vi "UTF8 Encoding to Unicode (UCS32).vi"(8 "error in":errorcluster, 9 "[UTF-8]":u8[](array[numeric])=[65, 226, 137, 162, 206, 145, 46, 237, 149, 156, 234, 189, 173, 236, 150, 180, 230, 151, 165, 230, 156, 172, 232, 170, 158, 240, 163, 142, 180] format="%.0x") -> (0 "error out":errorcluster, 1 "[UCS 32]":u32[](array[numeric]) format="%.0x", 4 "UCS 32":u32 format="%.0x")   [LabVIEW 2011]
doc: "Converts the given UTF-8 Encoded Unicode to UCS 32 Bit Representation of Unicode.\n\nUTF-8 is one of the Encodings to store the 21 bit Unicode numbers in a compact format.\n i.e. it stores the Unicode in one or more Byte sequences."
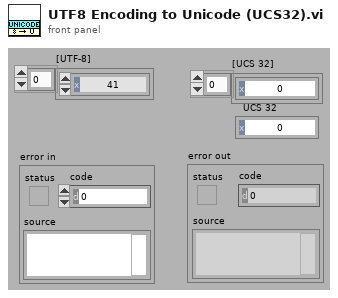
[diagram p1: front panel]
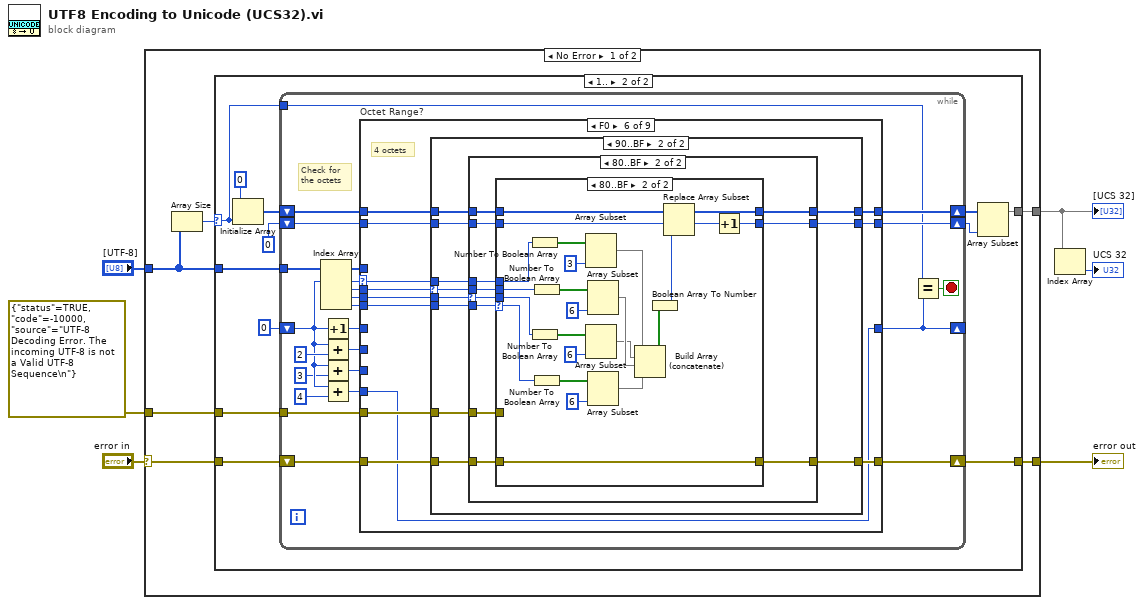
[diagram p0: block diagram]
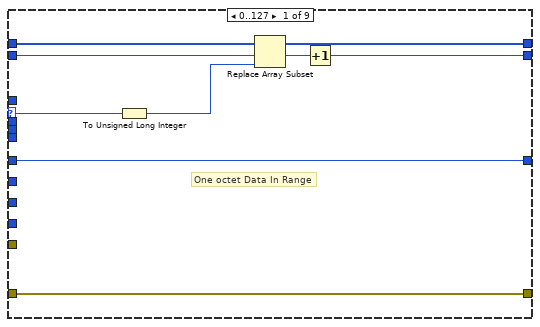
[diagram p3: hidden frame]
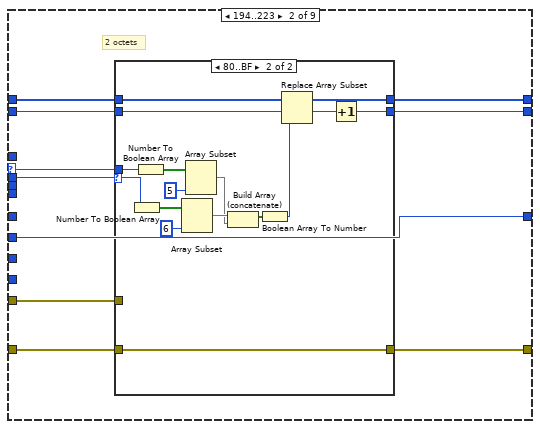
[diagram p4: hidden frame]
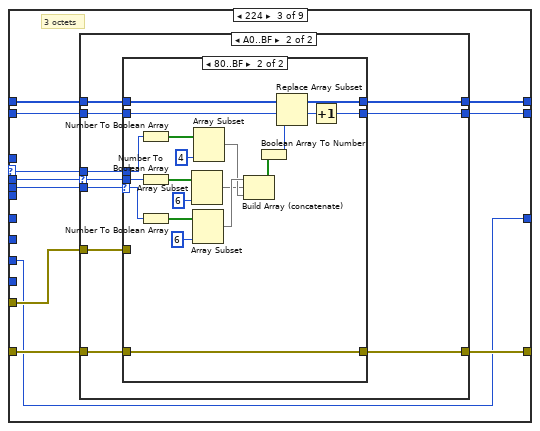
[diagram p6: hidden frame]
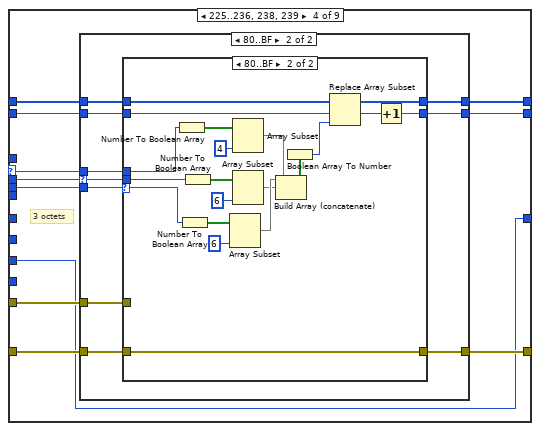
[diagram p9: hidden frame]
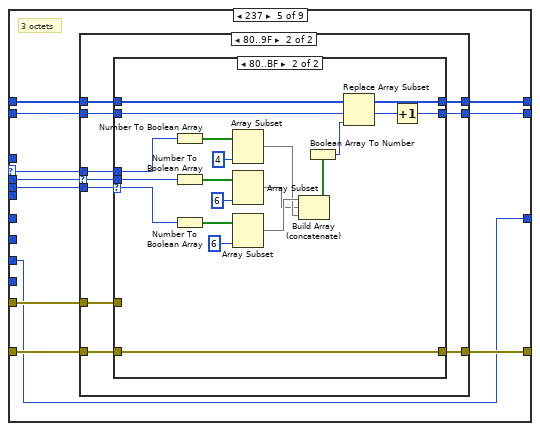
[diagram p12: hidden frame]
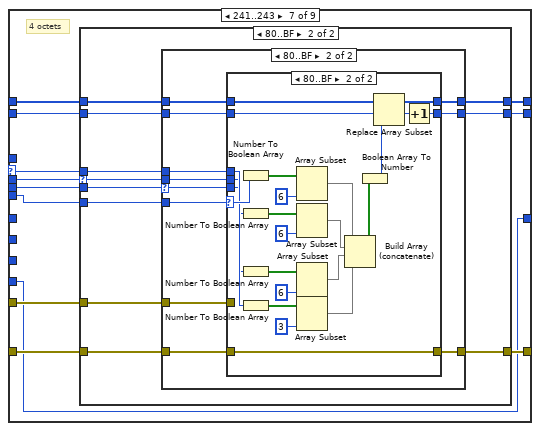
[diagram p18: hidden frame]
diagram:
  n1 = case shown="No Error" "error in" {
    selector: "error in" -> [w8 w427]
    tunnel: [w12 _] -> w3
    tunnel: "[UTF-8]" -> [w11 _]
    tunnel: [w9 w427] -> w5
    tunnel: errorcluster {"status"=TRUE, "code"=-10000, "source"="UTF-8 Decoding Error. The incoming UTF-8 is not a Valid UTF-8 Sequence\n"} ("error IO") -> [w7 _]
    frame No Error {
      n2 = Array Size(array=w11) -> (size(s)=w10:i32)
      n3 = case shown="1.." w10 {
        selector: w10 -> [_ w14]
        tunnel: [_ w19] -> w12
        tunnel: w11 -> [_ w16]
        tunnel: [w13 w24] -> w9
        tunnel: w8 -> [w13 w25]
        tunnel: w7 -> [_ w23]
        frame Default {
          # "No input \nNo output"
        }
        frame 1.. {
          n4 = Initialize Array(u32 0 ("UCS"), w14) -> (w22:u32[])
          n5 = while {
            shift-right: [w47] -> w20
            shift-left: w22 -> [w48]
            shift-right: [w45] -> w24
            shift-left: w25 -> [w46]
            tunnel: w23 -> [w44]
            shift-right: [w42] -> w18
            shift-left: 0 ("UCS") -> [w43]
            tunnel: w16 -> [w26]
            shift-right: [w37] -> _
            shift-left: 0 ("UCS") -> [w33]
            tunnel: w14 -> [w27]
            stop <- w36 stop-if-true
            # "Check for \nthe octets"
            n6 = Index Array(array=w26, index #1=w33) -> (element #1=w38:u8, element #2=w41:u8, element #3=w40:u8, element #4=w39:u8)  [unwired: 3 in]
            n7 = Increment(x=w33) -> (x+1=w35:i32)
            n8 = Add(x=w33, y=2) -> (x+y=w30:i32)
            n9 = Add(x=w33, y=3) -> (x+y=w29:i32)
            n10 = Add(x=w33, y=4) -> (x+y=w28:i32)
            n11 = case "Octet Range?" shown="F0" w38 {
              selector: w38 -> [w56 w66 w95 w141 w187 w234 w300 w366 _]
              tunnel: w26 -> [_ _ _ _ _ _ _ _ w426]
              tunnel: w48 -> [w54 w65 w94 w140 w186 w233 w299 w365 w424]
              tunnel: [w53 w64 w93 w139 w185 w232 w298 w364 w424] -> w47
              tunnel: w46 -> [w55 w63 w92 w137 w183 w230 w296 w362 _]
              tunnel: [w55 w62 w91 w138 w184 w231 w297 w363 w423] -> w45
              tunnel: w44 -> [_ w61 w90 w136 w182 w229 w295 w361 w423]
              tunnel: w43 -> [w51 w60 w88 w135 w181 w228 w294 w360 w422]
              tunnel: [w50 w59 w89 w134 w180 w227 w293 w359 w422] -> w42
              tunnel: w41 -> [_ w58 w86 w132 w178 w225 w292 w357 _]
              tunnel: w40 -> [_ _ w85 w131 w177 w224 w291 w356 _]
              tunnel: w39 -> [_ _ _ _ _ w223 w290 w355 _]
              tunnel: [w49 w57 w87 w133 w179 w226 w289 w358 w421] -> w37
              tunnel: w35 -> [w49 _ _ _ _ _ _ _ w421]
              tunnel: w30 -> [_ w57 _ _ _ _ _ _ _]
              tunnel: w29 -> [_ _ w87 w133 w179 _ _ _ _]
              tunnel: w28 -> [_ _ _ _ _ w226 w289 w358 _]
              frame 0..127 {
                # "One octet Data In Range"
                n12 = To Unsigned Long Integer(number=w56) -> (unsigned 32bit integer=w52:u32)
                n13 = Replace Array Subset(array=w54, new element=w52, index=w51) -> (w53:u32[])
                n14 = Increment(x=w51) -> (x+1=w50:i32)
              }
              frame 194..223 {
                # "2 octets"
                n15 = case shown="80..BF" w58 {
                  selector: w58 -> [_ w84]
                  tunnel: w66 -> [_ w83]
                  tunnel: w65 -> [w69 w74]
                  tunnel: [w69 w73] -> w64
                  tunnel: w63 -> [_ w75]
                  tunnel: [w68 w75] -> w62
                  tunnel: w61 -> [w68 _]
                  tunnel: w60 -> [w67 w71]
                  tunnel: [w67 w70] -> w59
                  frame Default {
                  }
                  frame 128..191 {
                    n16 = Number To Boolean Array(number=w84) -> (Boolean array=w82:bool[])
                    n17 = Number To Boolean Array(number=w83) -> (Boolean array=w81:bool[])
                    n18 = Array Subset(array=w82, length=6) -> (w78:bool[])  [unwired: 1 in]
                    n19 = Array Subset(array=w81, length=5) -> (w77:bool[])  [unwired: 1 in]
                    n20 = Build Array (concatenate)(w78, w77) -> (w76:bool[])
                    n21 = Boolean Array To Number(Boolean array=w76) -> (number=w72:u32)
                    n22 = Replace Array Subset(array=w74, new element=w72, index=w71) -> (w73:u32[])
                    n23 = Increment(x=w71) -> (x+1=w70:i32)
                  }
                }
              }
              frame 224 {
                # "3 octets"
                n24 = case shown="A0..BF" w86 {
                  selector: w86 -> [_ w105]
                  tunnel: w95 -> [_ w108]
                  tunnel: w94 -> [w98 w107]
                  tunnel: [w98 w106] -> w93
                  tunnel: w92 -> [_ w104]
                  tunnel: [w97 w103] -> w91
                  tunnel: w90 -> [w97 w102]
                  tunnel: [w96 w100] -> w89
                  tunnel: w88 -> [w96 w101]
                  tunnel: w85 -> [_ w99]
                  frame Default {
                  }
                  frame 160..191 {
                    n25 = case shown="80..BF" w99 {
                      selector: w99 -> [_ w130]
                      tunnel: w108 -> [_ w129]
                      tunnel: w107 -> [w111 w116]
                      tunnel: [w111 w115] -> w106
                      tunnel: w105 -> [_ w120]
                      tunnel: w104 -> [_ w117]
                      tunnel: [w110 w117] -> w103
                      tunnel: w102 -> [w110 _]
                      tunnel: w101 -> [w109 w113]
                      tunnel: [w109 w112] -> w100
                      frame Default {
                      }
                      frame 128..191 {
                        n26 = Number To Boolean Array(number=w129) -> (Boolean array=w127:bool[])
                        n27 = Number To Boolean Array(number=w120) -> (Boolean array=w121:bool[])
                        n28 = Number To Boolean Array(number=w130) -> (Boolean array=w128:bool[])
                        n29 = Array Subset(array=w121, length=6) -> (w118:bool[])  [unwired: 1 in]
                        n30 = Array Subset(array=w128, length=6) -> (w124:bool[])  [unwired: 1 in]
                        n31 = Array Subset(array=w127, length=4) -> (w119:bool[])  [unwired: 1 in]
                        n32 = Build Array (concatenate)(w124, w118, w119) -> (w123:bool[])
                        n33 = Boolean Array To Number(Boolean array=w123) -> (number=w114:u32)
                        n34 = Replace Array Subset(array=w116, new element=w114, index=w113) -> (w115:u32[])
                        n35 = Increment(x=w113) -> (x+1=w112:i32)
                      }
                    }
                  }
                }
              }
              frame 225..236, 238, 239 {
                # "3 octets"
                n36 = case shown="80..BF" w132 {
                  selector: w132 -> [_ w151]
                  tunnel: w141 -> [_ w154]
                  tunnel: w140 -> [w144 w153]
                  tunnel: [w144 w152] -> w139
                  tunnel: [w143 w150] -> w138
                  tunnel: w137 -> [_ w149]
                  tunnel: w136 -> [w143 w148]
                  tunnel: w135 -> [w142 w147]
                  tunnel: [w142 w146] -> w134
                  tunnel: w131 -> [_ w145]
                  frame Default {
                  }
                  frame 128..191 {
                    n37 = case shown="80..BF" w145 {
                      selector: w145 -> [_ w176]
                      tunnel: w154 -> [_ w175]
                      tunnel: w153 -> [w157 w162]
                      tunnel: [w157 w161] -> w152
                      tunnel: w151 -> [_ w166]
                      tunnel: [w156 w163] -> w150
                      tunnel: w149 -> [_ w163]
                      tunnel: w148 -> [w156 _]
                      tunnel: w147 -> [w155 w159]
                      tunnel: [w155 w158] -> w146
                      frame Default {
                      }
                      frame 128..191 {
                        n38 = Number To Boolean Array(number=w175) -> (Boolean array=w173:bool[])
                        n39 = Number To Boolean Array(number=w176) -> (Boolean array=w174:bool[])
                        n40 = Number To Boolean Array(number=w166) -> (Boolean array=w167:bool[])
                        n41 = Array Subset(array=w174, length=6) -> (w170:bool[])  [unwired: 1 in]
                        n42 = Array Subset(array=w173, length=4) -> (w165:bool[])  [unwired: 1 in]
                        n43 = Array Subset(array=w167, length=6) -> (w164:bool[])  [unwired: 1 in]
                        n44 = Build Array (concatenate)(w170, w164, w165) -> (w169:bool[])
                        n45 = Boolean Array To Number(Boolean array=w169) -> (number=w160:u32)
                        n46 = Replace Array Subset(array=w162, new element=w160, index=w159) -> (w161:u32[])
                        n47 = Increment(x=w159) -> (x+1=w158:i32)
                      }
                    }
                  }
                }
              }
              frame 237 {
                # "3 octets"
                n48 = case shown="80..9F" w178 {
                  selector: w178 -> [_ w197]
                  tunnel: w187 -> [_ w200]
                  tunnel: w186 -> [w190 w199]
                  tunnel: [w190 w198] -> w185
                  tunnel: [w189 w196] -> w184
                  tunnel: w183 -> [_ w195]
                  tunnel: w182 -> [w189 w194]
                  tunnel: w181 -> [w188 w193]
                  tunnel: [w188 w192] -> w180
                  tunnel: w177 -> [_ w191]
                  frame Default {
                  }
                  frame 128..159 {
                    n49 = case shown="80..BF" w191 {
                      selector: w191 -> [_ w222]
                      tunnel: w200 -> [_ w221]
                      tunnel: w199 -> [w203 w208]
                      tunnel: [w203 w207] -> w198
                      tunnel: w197 -> [_ w212]
                      tunnel: [w202 w209] -> w196
                      tunnel: w195 -> [_ w209]
                      tunnel: w194 -> [w202 _]
                      tunnel: w193 -> [w201 w205]
                      tunnel: [w201 w204] -> w192
                      frame Default {
                      }
                      frame 128..191 {
                        n50 = Number To Boolean Array(number=w221) -> (Boolean array=w219:bool[])
                        n51 = Number To Boolean Array(number=w212) -> (Boolean array=w213:bool[])
                        n52 = Number To Boolean Array(number=w222) -> (Boolean array=w220:bool[])
                        n53 = Array Subset(array=w219, length=4) -> (w211:bool[])  [unwired: 1 in]
                        n54 = Array Subset(array=w213, length=6) -> (w210:bool[])  [unwired: 1 in]
                        n55 = Array Subset(array=w220, length=6) -> (w216:bool[])  [unwired: 1 in]
                        n56 = Build Array (concatenate)(w216, w210, w211) -> (w215:bool[])
                        n57 = Boolean Array To Number(Boolean array=w215) -> (number=w206:u32)
                        n58 = Replace Array Subset(array=w208, new element=w206, index=w205) -> (w207:u32[])
                        n59 = Increment(x=w205) -> (x+1=w204:i32)
                      }
                    }
                  }
                }
              }
              frame 240 {
                # "4 octets"
                n60 = case shown="90..BF" w225 {
                  selector: w225 -> [_ w245]
                  tunnel: w234 -> [_ w248]
                  tunnel: w233 -> [w237 w247]
                  tunnel: [w237 w246] -> w232
                  tunnel: [w236 w244] -> w231
                  tunnel: w230 -> [_ w243]
                  tunnel: w229 -> [w236 w242]
                  tunnel: w228 -> [w235 w241]
                  tunnel: [w235 w240] -> w227
                  tunnel: w224 -> [_ w239]
                  tunnel: w223 -> [_ w238]
                  frame Default {
                  }
                  frame 144..191 {
                    n61 = case shown="80..BF" w239 {
                      selector: w239 -> [_ w258]
                      tunnel: w248 -> [_ w262]
                      tunnel: w247 -> [w251 w261]
                      tunnel: [w251 w260] -> w246
                      tunnel: w245 -> [_ w259]
                      tunnel: [w250 w257] -> w244
                      tunnel: w243 -> [_ w256]
                      tunnel: w242 -> [w250 w255]
                      tunnel: w241 -> [w249 w254]
                      tunnel: [w249 w253] -> w240
                      tunnel: w238 -> [_ w252]
                      frame Default {
                      }
                      frame 128..191 {
                        n62 = case shown="80..BF" w252 {
                          selector: w252 -> [_ w288]
                          tunnel: w262 -> [_ w287]
                          tunnel: w261 -> [w265 w281]
                          tunnel: [w265 w280] -> w260
                          tunnel: w259 -> [_ w277]
                          tunnel: w258 -> [_ w273]
                          tunnel: [w264 w269] -> w257
                          tunnel: w256 -> [_ w269]
                          tunnel: w255 -> [w264 _]
                          tunnel: w254 -> [w263 w267]
                          tunnel: [w263 w266] -> w253
                          frame Default {
                          }
                          frame 128..191 {
                            n63 = Number To Boolean Array(number=w287) -> (Boolean array=w285:bool[])
                            n64 = Number To Boolean Array(number=w273) -> (Boolean array=w272:bool[])
                            n65 = Number To Boolean Array(number=w277) -> (Boolean array=w278:bool[])
                            n66 = Number To Boolean Array(number=w288) -> (Boolean array=w286:bool[])
                            n67 = Array Subset(array=w285, length=3) -> (w276:bool[])  [unwired: 1 in]
                            n68 = Array Subset(array=w272, length=6) -> (w271:bool[])  [unwired: 1 in]
                            n69 = Array Subset(array=w278, length=6) -> (w275:bool[])  [unwired: 1 in]
                            n70 = Array Subset(array=w286, length=6) -> (w270:bool[])  [unwired: 1 in]
                            n71 = Build Array (concatenate)(w270, w271, w275, w276) -> (w282:bool[])
                            n72 = Boolean Array To Number(Boolean array=w282) -> (number=w268:u32)
                            n73 = Replace Array Subset(array=w281, new element=w268, index=w267) -> (w280:u32[])
                            n74 = Increment(x=w267) -> (x+1=w266:i32)
                          }
                        }
                      }
                    }
                  }
                }
              }
              frame 241..243 {
                # "4 octets"
                n75 = case shown="80..BF" w292 {
                  selector: w292 -> [_ w311]
                  tunnel: w300 -> [_ w314]
                  tunnel: w299 -> [w303 w313]
                  tunnel: [w303 w312] -> w298
                  tunnel: [w302 w310] -> w297
                  tunnel: w296 -> [_ w309]
                  tunnel: w295 -> [w302 w308]
                  tunnel: w294 -> [w301 w307]
                  tunnel: [w301 w306] -> w293
                  tunnel: w291 -> [_ w305]
                  tunnel: w290 -> [_ w304]
                  frame Default {
                  }
                  frame 128..191 {
                    n76 = case shown="80..BF" w305 {
                      selector: w305 -> [_ w324]
                      tunnel: w314 -> [_ w328]
                      tunnel: w313 -> [w317 w327]
                      tunnel: [w317 w326] -> w312
                      tunnel: w311 -> [_ w325]
                      tunnel: [w316 w323] -> w310
                      tunnel: w309 -> [_ w322]
                      tunnel: w308 -> [w316 w321]
                      tunnel: w307 -> [w315 w320]
                      tunnel: [w315 w319] -> w306
                      tunnel: w304 -> [_ w318]
                      frame Default {
                      }
                      frame 128..191 {
                        n77 = case shown="80..BF" w318 {
                          selector: w318 -> [_ w354]
                          tunnel: w328 -> [_ w353]
                          tunnel: w327 -> [w331 w336]
                          tunnel: [w331 w335] -> w326
                          tunnel: w325 -> [_ w345]
                          tunnel: w324 -> [_ w341]
                          tunnel: [w330 w337] -> w323
                          tunnel: w322 -> [_ w337]
                          tunnel: w321 -> [w330 _]
                          tunnel: w320 -> [w329 w333]
                          tunnel: [w329 w332] -> w319
                          frame Default {
                          }
                          frame 128..191 {
                            n78 = Number To Boolean Array(number=w354) -> (Boolean array=w352:bool[])
                            n79 = Number To Boolean Array(number=w341) -> (Boolean array=w340:bool[])
                            n80 = Number To Boolean Array(number=w345) -> (Boolean array=w346:bool[])
                            n81 = Number To Boolean Array(number=w353) -> (Boolean array=w351:bool[])
                            n82 = Array Subset(array=w352, length=6) -> (w338:bool[])  [unwired: 1 in]
                            n83 = Array Subset(array=w340, length=6) -> (w339:bool[])  [unwired: 1 in]
                            n84 = Array Subset(array=w346, length=6) -> (w343:bool[])  [unwired: 1 in]
                            n85 = Array Subset(array=w351, length=3) -> (w344:bool[])  [unwired: 1 in]
                            n86 = Build Array (concatenate)(w338, w339, w343, w344) -> (w348:bool[])
                            n87 = Boolean Array To Number(Boolean array=w348) -> (number=w334:u32)
                            n88 = Replace Array Subset(array=w336, new element=w334, index=w333) -> (w335:u32[])
                            n89 = Increment(x=w333) -> (x+1=w332:i32)
                          }
                        }
                      }
                    }
                  }
                }
              }
              frame 244 {
                # "4 octets"
                n90 = case shown="80..8F" w357 {
                  selector: w357 -> [_ w377]
                  tunnel: w366 -> [_ w380]
                  tunnel: w365 -> [w369 w379]
                  tunnel: [w369 w378] -> w364
                  tunnel: [w368 w376] -> w363
                  tunnel: w362 -> [_ w375]
                  tunnel: w361 -> [w368 w374]
                  tunnel: w360 -> [w367 w373]
                  tunnel: [w367 w372] -> w359
                  tunnel: w356 -> [_ w371]
                  tunnel: w355 -> [_ w370]
                  frame Default {
                  }
                  frame 128..143 {
                    n91 = case shown="80..BF" w371 {
                      selector: w371 -> [_ w390]
                      tunnel: w380 -> [_ w394]
                      tunnel: w379 -> [w383 w393]
                      tunnel: [w383 w392] -> w378
                      tunnel: w377 -> [_ w391]
                      tunnel: [w382 w389] -> w376
                      tunnel: w375 -> [_ w388]
                      tunnel: w374 -> [w382 w387]
                      tunnel: w373 -> [w381 w386]
                      tunnel: [w381 w385] -> w372
                      tunnel: w370 -> [_ w384]
                      frame Default {
                      }
                      frame 128..191 {
                        n92 = case shown="80..BF" w384 {
                          selector: w384 -> [_ w420]
                          tunnel: w394 -> [_ w419]
                          tunnel: w393 -> [w397 w402]
                          tunnel: [w397 w401] -> w392
                          tunnel: w391 -> [_ w411]
                          tunnel: w390 -> [_ w407]
                          tunnel: [w396 w403] -> w389
                          tunnel: w388 -> [_ w403]
                          tunnel: w387 -> [w396 _]
                          tunnel: w386 -> [w395 w399]
                          tunnel: [w395 w398] -> w385
                          frame Default {
                          }
                          frame 128..191 {
                            n93 = Number To Boolean Array(number=w419) -> (Boolean array=w417:bool[])
                            n94 = Number To Boolean Array(number=w411) -> (Boolean array=w412:bool[])
                            n95 = Number To Boolean Array(number=w407) -> (Boolean array=w406:bool[])
                            n96 = Number To Boolean Array(number=w420) -> (Boolean array=w418:bool[])
                            n97 = Array Subset(array=w417, length=3) -> (w410:bool[])  [unwired: 1 in]
                            n98 = Array Subset(array=w412, length=6) -> (w409:bool[])  [unwired: 1 in]
                            n99 = Array Subset(array=w406, length=6) -> (w405:bool[])  [unwired: 1 in]
                            n100 = Array Subset(array=w418, length=6) -> (w404:bool[])  [unwired: 1 in]
                            n101 = Build Array (concatenate)(w404, w405, w409, w410) -> (w414:bool[])
                            n102 = Boolean Array To Number(Boolean array=w414) -> (number=w400:u32)
                            n103 = Replace Array Subset(array=w402, new element=w400, index=w399) -> (w401:u32[])
                            n104 = Increment(x=w399) -> (x+1=w398:i32)
                          }
                        }
                      }
                    }
                  }
                }
              }
              frame Default {
                # "One octect Out of Range"
                n105 = Delete From Array(array=w426, index=0) -> ()  [unwired: 1 in, 2 out]
              }
            }
            n106 = Equal?(x=w27, y=w37) -> (x = y?=w36:bool)
          }
          n107 = Array Subset(array=w20, length=w18) -> (w19:u32[])  [unwired: 1 in]
        }
      }
    }
    frame Error {
      # "Do nothing on incoming Error"
    }
  }
  "[UCS 32]" <- w3
  "error out" <- w5
  n108 = Index Array(array=w3) -> (element=→"UCS 32":u32)  [unwired: 1 in]
